vi "Log State.vi"(8 "error in (no error)":errorcluster, 9 "line text":string, 10 "line tag":string, 11 "Logging Thread in":refnum<class "Logging Thread.lvclass">) -> (0 "error out":errorcluster, 3 "Logging Thread out":refnum<class "Logging Thread.lvclass">)   [LabVIEW 2019, in "DSF Core.lvlib" / "Logging Thread.lvclass"]
uses:
  Logging Thread.lvclass
  Logging Thread.lvclass/Logging Thread.ctl
  <vilib>/Utility/High Resolution Relative Seconds.vi
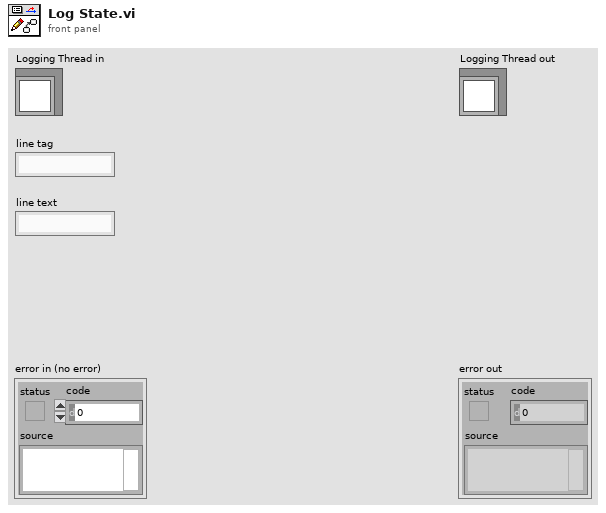
[diagram p1: front panel]
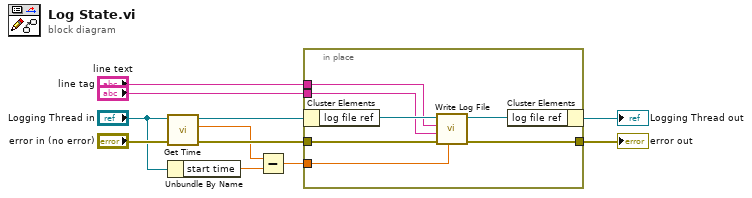
[diagram p0: block diagram]
diagram:
  n1 = call "Get Time.vi"("error in (no error)"="error in (no error)", "Logging Thread in"="Logging Thread in") -> ("error out"=w6:errorcluster, "time"=w4:dbl, "Logging Thread out"=w5:refnum<class "Logging Thread.lvclass">)  [unwired: 7 in]
  n2 = Unbundle By Name("Logging Thread in") -> ("start time"=w3:dbl)
  n3 = Subtract(x=w4, y=w3) -> (x-y=w1:dbl)
  n4 = in-place {
    in-place-border: w6 -> [w16]
    in-place-border: [w15] -> w11
    in-place-border: "line text" -> [w14]
    in-place-border: "line tag" -> [w13]
    in-place-border: w1 -> [w12]
    n5 = in-place-cluster #1(w5) -> ("log file ref"=w18:refnum<file>)
    n6 = call "Write Log File.vi"("time"=w12, "error in (no error)"=w16, "line text"=w14, "line tag"=w13, "file refnum in"=w18) -> ("error out"=w15:errorcluster, "file refnum out"=w17:refnum<file>)  [unwired: 5 in]
    n7 = in-place-cluster #1("log file ref"=w17) -> (→"Logging Thread out":refnum<class "Logging Thread.lvclass">)
  }
  "error out" <- w11
